vi "Modularized-3LOOPs-w-EH-Main.vi"() -> ()   [LabVIEW 2021]
uses:
  _Core/Core-CtrlRefs.ctl
panel:
  in  "PauseDAQ":bool
  out "Chart":dbl(graph)
  in  "Ctrl-Refs":T1
  in  "Exit":bool
  in  "StartDAQ":bool
  # "Send Start/Pause DAQ\nmessage to DAQ module\nto control the DAQ loop.\n\nUse Char t Reference to\nupdate the GUI from DAQ\nloop directly."
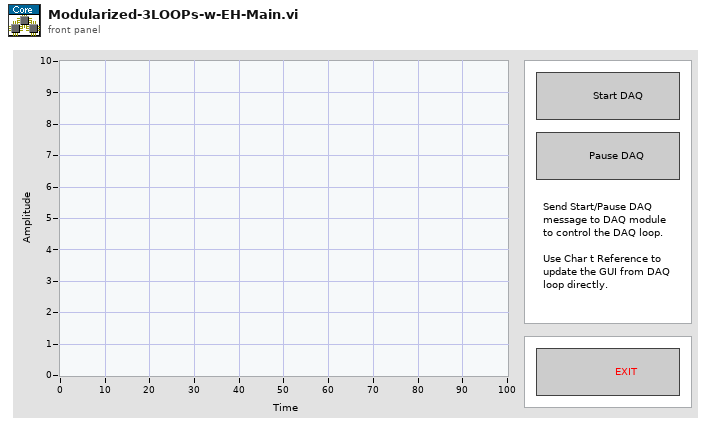
[diagram p1: front panel]
types:
  T1 = typedef "Core-CtrlRefs.ctl" = cluster{"Bool Refnum":refnum<vi>, "WFChart Refnum":refnum<vi>}
  T2 = cluster{"GUI::Initialize":refnum<user-event>, "GUI::User1":refnum<user-event>}
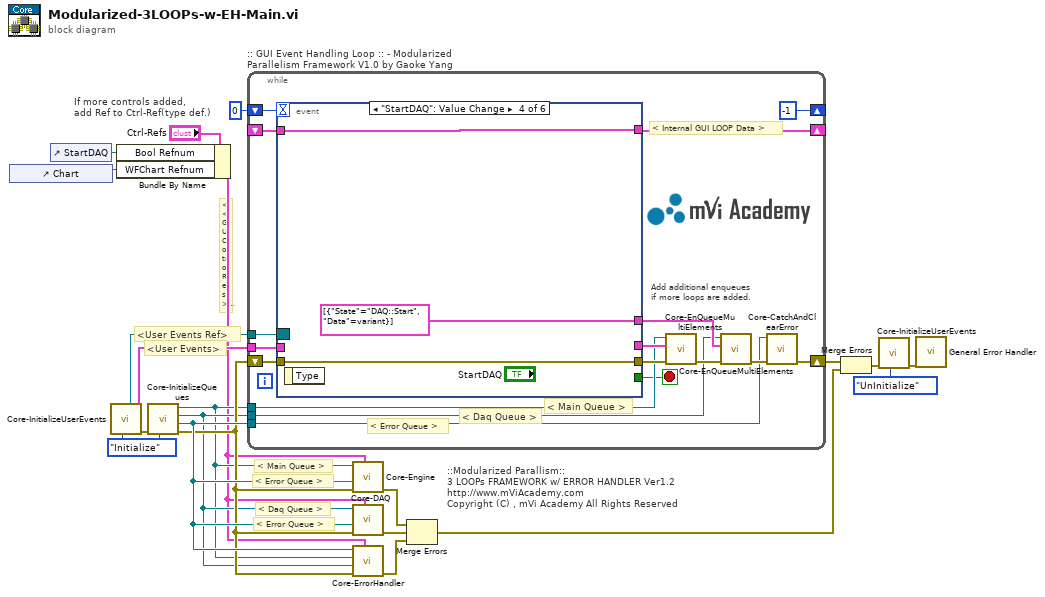
[diagram p0: block diagram]
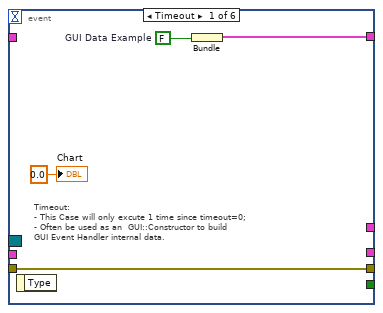
[diagram p2: hidden frame]
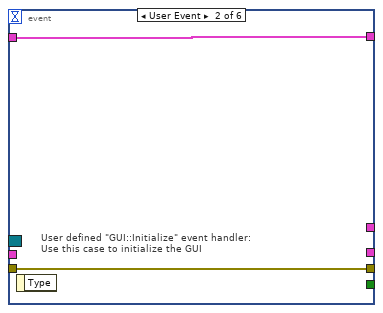
[diagram p3: hidden frame]
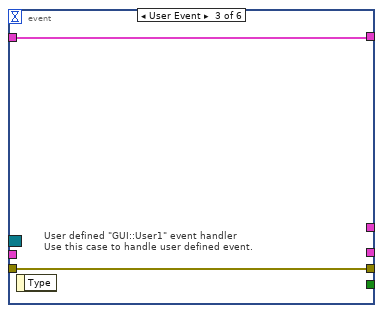
[diagram p4: hidden frame]
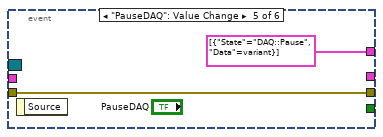
[diagram p5: hidden frame]
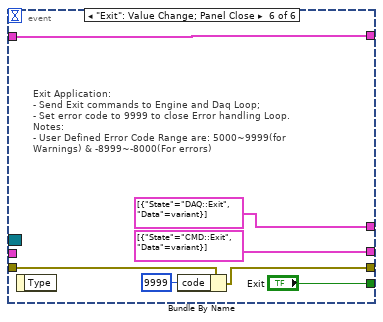
[diagram p6: hidden frame]
diagram:
  w18 = enum16{"Initialize", "UnInitialize"}."Initialize" ("Cmd(Initialize)")
  # "< Error Queue >"
  # "< Daq Queue >"
  # "< Error Queue >"
  # "< Main Queue >"
  # "If more controls added, \nadd Ref to Ctrl-Ref(type def.)"
  # "<< GUI Control Refs >>"
  # "<User Events>"
  # "<User Events Ref>"
  # "::Modularized Parallism::\n3 LOOPs FRAMEWORK w/ ERROR HANDLER Ver1.2\nhttp://www.mViAcademy.com\nCopyright (C) , mVi Academy All Rights Reserved"
  n1 = control-ref of="Chart"() -> (w1:refnum<vi>)
  n2 = control-ref of="StartDAQ"() -> (w6:refnum<vi>)
  n3 = call "Core-InitializeUserEvents.vi"("Cmd(Initialize)"=w18) -> ("ErrO"=w19:errorcluster, "User Events"=w17:T2, "User Events\nRefnum"=w9:refnum<event-registration>)  [unwired: 8 in]
  n4 = Bundle By Name(cluster="Ctrl-Refs", "Bool Refnum"=w6, "WFChart Refnum"=w1) -> (w7:T1)
  n5 = call "Core-InitializeQueues.vi"("Cmd(Initialize)"=w18, "ErrI(No Error)"=w19) -> ("ErrO"=w12:errorcluster, "ErrQRef"=w13:refnum<queue>, "DaqQRef"=w11:refnum<queue>, "MainQRef"=w10:refnum<queue>)  [unwired: 6 in]
  n6 = while ":: GUI Event Handling Loop :: - Modularized Parallelism Framework V1.0 by Gaoke Yang" {
    tunnel: w10 -> [w34]
    shift-right: [w28] -> w20
    shift-left: w12 -> [w38]
    tunnel: w11 -> [w31]
    tunnel: w17 -> [w22]
    tunnel: w13 -> [w29]
    tunnel: w9 -> [w23]
    shift-right: [-1] -> _
    shift-left: 0 -> [w26]
    shift-right: [w25] -> _
    shift-left: _ -> [w24]
    stop <- w32 stop-if-true
    # "< Internal GUI LOOP Data >"
    # "Add additional enqueues \nif more loops are added."
    # "< Main Queue >"
    # "< Error Queue >"
    # "< Daq Queue >"
    n7 = event shown="[3] \"StartDAQ\": Value Change" {
      selector: w23 -> [_ _ _ _ _ _]
      dyn-events: _ -> [_ _ _ _ _ _]
      timeout: w26 -> [_ _ _ _ _ _]
      tunnel: [_ _ _ _ _ "Exit"] -> w32
      tunnel: w38 -> [w42 w44 w46 w49 w51 w55]
      tunnel: [w42 w44 w46 w49 w51 w54] -> w36
      tunnel: [_ _ _ _ _ cluster{"State":string, "Data":variant}[] [{"State"="CMD::Exit", "Data"=variant}]] -> w37
      tunnel: [_ _ _ cluster{"State":string, "Data":variant}[] [{"State"="DAQ::Start", "Data"=variant}] cluster{"State":string, "Data":variant}[] [{"State"="DAQ::Pause", "Data"=variant}] cluster{"State":string, "Data":variant}[] [{"State"="DAQ::Exit", "Data"=variant}]] -> w33
      tunnel: [w40 w43 w45 w47 _ w52] -> w25
      tunnel: w24 -> [_ w43 w45 w47 _ w52]
      tunnel: w22 -> [_ _ _ _ _ _]
      event Timeout {
        w41 = FALSE  # GUI Data Example
        # "Timeout:\n- This Case will only excute 1 time since timeout=0;\n- Often be used as an  GUI::Constructor to build\nGUI Event Handler internal data."
        n8 = event-data() -> ()  [unwired: 2 out]
        n9 = Bundle("GUI Data Example"=w41) -> (w40:cluster{"GUI Data Example":bool})  [unwired: 1 in]
        "Chart" <- 0.0 ("Chart")
      }
      event User Event {
        # "User defined \"GUI::Initialize\" event handler:\nUse this case to initialize the GUI"
        n10 = event-data() -> ()  [unwired: 2 out]
      }
      event User Event {
        # "User defined \"GUI::User1\" event handler\nUse this case to handle user defined event."
        n11 = event-data() -> ()  [unwired: 2 out]
      }
      event "StartDAQ": Value Change {
        n12 = event-data() -> ()  [unwired: 2 out]
      }
      event "PauseDAQ": Value Change {
        n13 = event-data() -> ()  [unwired: 2 out]
      }
      event "Exit": Value Change; Panel Close {
        # "Exit Application:\n- Send Exit commands to Engine and Daq Loop;\n- Set error code to 9999 to close Error handling Loop.\nNotes:\n- User Defined Error Code Range are: 5000~9999(for Warnings) & -8999~-8000(For errors)"
        n14 = event-data() -> ()  [unwired: 2 out]
        n15 = Bundle By Name(cluster=w55, "code"=9999) -> (w54:errorcluster)
      }
    }
    n16 = call "Core-EnQueueMultiElements.vi"("ErrorIn"=w36, "CmdArray"=w37, "QRefIn"=w34) -> ("ErrorOut"=w35:errorcluster)  [unwired: 8 in]
    n17 = call "Core-EnQueueMultiElements.vi"("ErrorIn"=w35, "CmdArray"=w33, "QRefIn"=w31) -> ("ErrorOut"=w30:errorcluster)  [unwired: 8 in]
    n18 = call "Core-CatchAndClearError.vi"("Err-I"=w30, "ErrQ-I"=w29) -> ("Err-O"=w28:errorcluster)  [unwired: 9 in]
  }
  n19 = call "Core-Engine.vi"("Ctrl-Refs"=w7, "Err-I"=w12, "ErrQRef"=w13, "MainQ-I"=w10) -> ("Err-O"=w5:errorcluster)  [unwired: 7 in]
  n20 = call "Core-DAQ.vi"("Ctrl-Refs"=w7, "Err-I"=w12, "ErrQRef"=w13, "DaqQ-I"=w11) -> ("Err-O"=w4:errorcluster)  [unwired: 7 in]
  n21 = call "Core-ErrorHandler.vi"("Ctrl-Refs"=w7, "Err-I"=w12, "DaqQ-I"=w11, "MainQ-I"=w10, "ErrQ-I"=w13) -> ("Err-O"=w3:errorcluster)  [unwired: 6 in]
  n22 = Merge Errors(w5, w4, w3) -> (w2:errorcluster)
  n23 = Merge Errors(w20, w2) -> (w15:errorcluster)
  n24 = call "Core-InitializeUserEvents.vi"("Cmd(Initialize)"=enum16{"Initialize", "UnInitialize"}."UnInitialize", "ErrI(No Error)"=w15) -> ("ErrO"=w14:errorcluster)  [unwired: 7 in, 2 out]
  n25 = call <vilib>:"General Error Handler.vi"("error in (no error)"=w14) -> ()  [unwired: 10 in, 5 out]
